vi "Set Select Platform Event.vi"(8 "error in (no error)":errorcluster, 10 "Select Platform":refnum<user-event>, 11 "PlatformListPanel in":refnum<class "PlatformListPanel.lvclass">) -> (0 "error out":errorcluster, 3 "PlatformListPanel out":refnum<class "PlatformListPanel.lvclass">)   [LabVIEW 2020, in "PicoG-App.lvlib" / "PlatformListPanel.lvclass"]
uses:
  PlatformListPanel.lvclass
  PlatformListPanel.lvclass/PlatformListPanel.ctl
  Builds/picoG/ppl/PicoG-Core.lvlibp/PicoG-Processor/PicoG-Core/DeployPlatform/Platform.lvclass
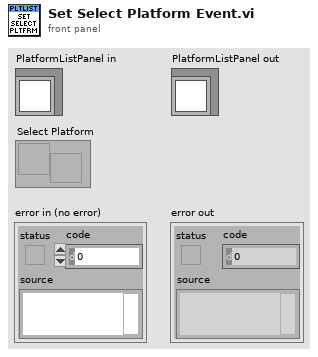
[diagram p1: front panel]
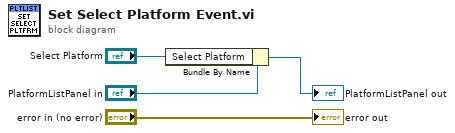
[diagram p0: block diagram]
diagram:
  n1 = Bundle By Name(cluster="PlatformListPanel in", "Select Platform"="Select Platform") -> (→"PlatformListPanel out":refnum<class "PlatformListPanel.lvclass">)
  "error out" <- "error in (no error)"
